vi "Configure Trigger (Setup Hold).vi"(0 "VISA resource name":refnum<visa-resource-name>, 1 "Data Type (0: H)":i32(ring) items=["H", "L"], 2 "Setup Time (5E-5 s)":dbl=5e-05, 5 "Data Source (1: Channel 1)":i32(ring)=1 items=["Channel 1"=1, "Channel 2"=2, "Channel 3"=3, "Channel 4"=4], 7 "Clock Source (1: Channel 1)":i32(ring)=2 items=["Channel 1"=1, "Channel 2"=2, "Channel 3"=3, "Channel 4"=4], 9 "Edge Type (0: Positive)":i32(ring) items=["Positive", "Negative"], 11 "error in (no error)":errorcluster, 12 "Hold Type (0: Setup)":i32(ring) items=["Setup", "Hold"], 13 "Hold Time (5E-8 s)":dbl=5e-08) -> (4 "VISA resource name out":refnum<visa-resource-name>, 15 "error out":errorcluster)   [LabVIEW 2015, in "ZhiYuan ZDS Series for TCP.lvlib"]
doc: "Configures the setting for setup hold setting.\n\nNote: This VI is only applicable for DS 2000 Series."
uses:
  ZhiYuan ZDS Series for TCP.lvlib
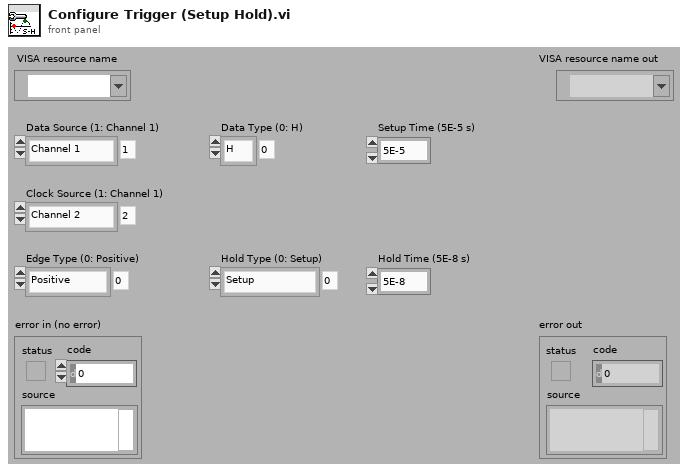
[diagram p1: front panel]
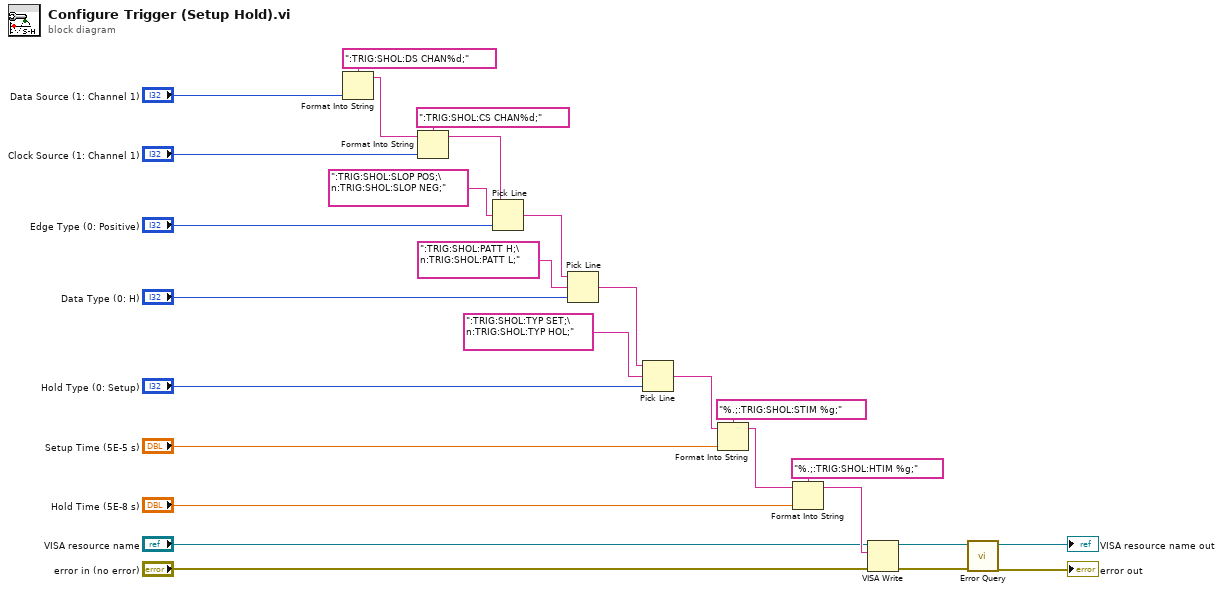
[diagram p0: block diagram]
diagram:
  n1 = Format Into String(format string=":TRIG:SHOL:DS CHAN%d;", "Data Source (1: Channel 1)") -> (resulting string=w25:string)  [unwired: 2 in, 1 out]
  n2 = Format Into String(format string=":TRIG:SHOL:CS CHAN%d;", initial string=w25, "Clock Source (1: Channel 1)") -> (resulting string=w20:string)  [unwired: 1 in, 1 out]
  n3 = Pick Line(string ("")=w20, multi-line string=":TRIG:SHOL:SLOP POS;\n:TRIG:SHOL:SLOP NEG;", line index="Edge Type (0: Positive)") -> (output string=w17:string)
  n4 = Pick Line(string ("")=w17, multi-line string=":TRIG:SHOL:PATT H;\n:TRIG:SHOL:PATT L;", line index="Data Type (0: H)") -> (output string=w14:string)
  n5 = Pick Line(string ("")=w14, multi-line string=":TRIG:SHOL:TYP SET;\n:TRIG:SHOL:TYP HOL;", line index="Hold Type (0: Setup)") -> (output string=w13:string)
  n6 = Format Into String(format string="%.;:TRIG:SHOL:STIM %g;", initial string=w13, "Setup Time (5E-5 s)") -> (resulting string=w10:string)  [unwired: 1 in, 1 out]
  n7 = Format Into String(format string="%.;:TRIG:SHOL:HTIM %g;", initial string=w10, "Hold Time (5E-8 s)") -> (resulting string=w7:string)  [unwired: 1 in, 1 out]
  n8 = VISA Write(VISA resource name="VISA resource name", write buffer=w7, error in (no error)="error in (no error)") -> (VISA resource name out=w4:refnum<visa-resource-name>, error out=w3:errorcluster)  [unwired: 1 out]
  n9 = call "Error Query.vi"("error in (no error)"=w3, "VISA resource name"=w4) -> ("error out"=→"error out":errorcluster, "VISA resource name out"=→"VISA resource name out":refnum<visa-resource-name>)  [unwired: 6 in, 2 out]
